vi "VXM-MoveAllThreeSubSystemsToHome.vi"(8 "error in (no error)":errorcluster, 9 "Move-Abs":T3={"Move Type"="AllHomeMove", "Positions"=[], "Position (Antenna or Raster)"=0, "Polarization"=0} {"Polarization" items=["Vertical", "Horizontal"]}, 11 "Message que":T4) -> (0 "error out":errorcluster)   [LabVIEW 2018]
uses:
  Support/MessageQue/MessageQue.ctl
  Support/MessageQue/MessageCluster.ctl
  singleAxisMoveDef.ctl
  mmWaveAxis.ctl
  Support/MessageQue/MessageQue.lvlib
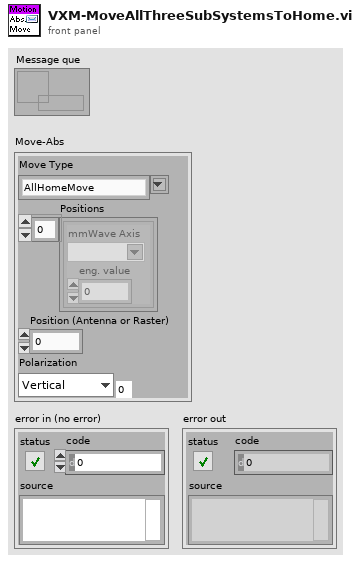
[diagram p1: front panel]
types:
  T1 = typedef "singleAxisMoveDef.ctl" = cluster{"mmWave Axis":T2, "eng. value":dbl}
  T2 = typedef "mmWaveAxis.ctl" = string
  T3 = cluster{"Move Type":string, "Positions":T1[], "Position (Antenna or Raster)":i32, "Polarization":u16}
  T4 = typedef "MessageQue.lvlib/MessageQue.ctl" = refnum<queue>
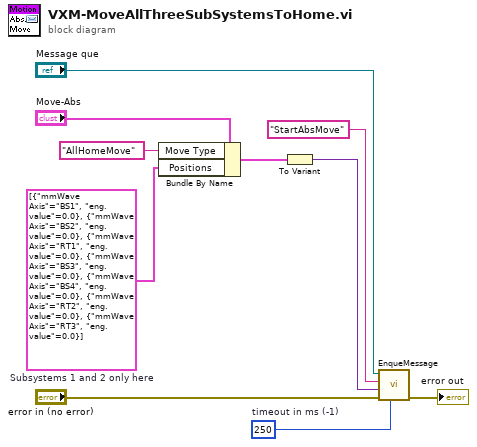
[diagram p0: block diagram]
diagram:
  w1 = T1[] [{"mmWave Axis"="BS1", "eng. value"=0.0}, {"mmWave Axis"="BS2", "eng. value"=0.0}, {"mmWave Axis"="RT1", "eng. value"=0.0}, {"mmWave Axis"="BS3", "eng. value"=0.0}, {"mmWave Axis"="BS4", "eng. value"=0.0}, {"mmWave Axis"="RT2", "eng. value"=0.0}, {"mmWave Axis"="RT3", "eng. value"=0.0}]  # Subsystems 1 and 2 only here
  w9 = 250  # timeout in ms (-1)
  n1 = Bundle By Name(cluster="Move-Abs", "Move Type"="AllHomeMove", "Positions"=w1) -> (w3:T3)
  n2 = To Variant(anything=w3) -> (Variant=w10:variant)
  n3 = call "EnqueMessage.vi"("timeout in ms (-1)"=w9, "error in"="error in (no error)", "Message Payload"=w10, "Message Command"="StartAbsMove", "Message que"="Message que") -> ("error out"=→"error out":errorcluster)  [unwired: 5 in, 1 out]
